vi "Init Async State Vars.vi"(8 "Error in":errorcluster, 10 "Async Parameters":T4) -> (0 "Error out":errorcluster, 3 "Async State Vars":T1)   [LabVIEW 2014, in "Waveform-Processing-Custom-Device Engine.lvlib"]
uses:
  Waveform-Processing-Custom-Device Engine.lvlib
  Types/Async Parameters.ctl
  Types/Async FIFOs.ctl
  <vilib>/NI Veristand/Custom Device API/Waveform Data Reference.ctl
  Types/Async State Vars.ctl
  <vilib>/NI Veristand/Custom Device Waveform API/Single Waveform Read (DBL)/Single Waveform Read (DBL).lvclass
  <vilib>/NI Veristand/Custom Device Waveform API/Single Waveform Write (DBL)/Single Waveform Write (DBL).lvclass
  <vilib>/NI Veristand/Custom Device API/Custom Device API.lvlib
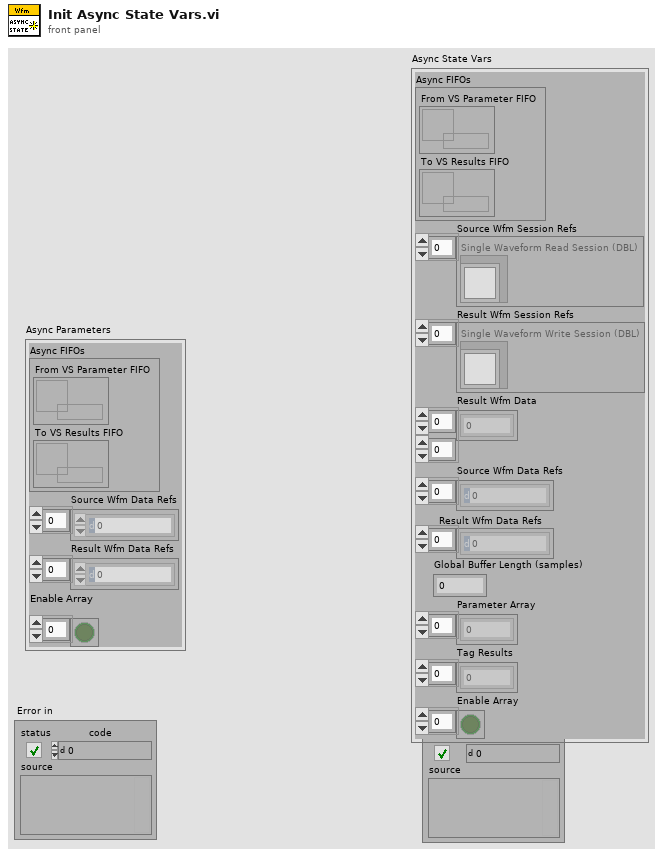
[diagram p1: front panel]
types:
  T1 = typedef "Waveform-Processing-Custom-Device Engine.lvlib/Async State Vars.ctl" = cluster{"Async FIFOs":T2, "Source Wfm Session Refs":refnum<class "Single Waveform Read (DBL).lvclass">[], "Result Wfm Session Refs":refnum<class "Single Waveform Write (DBL).lvclass">[], "Result Wfm Data":dbl[][], "Source Wfm Data Refs":T3[], "Result Wfm Data Refs":T3[], "Global Buffer Length (samples)":dbl, "Parameter Array":dbl[], "Tag Results":dbl[], "Enable Array":bool[]}
  T2 = typedef "Waveform-Processing-Custom-Device Engine.lvlib/Async FIFOs.ctl" = cluster{"From VS Parameter FIFO":refnum<k33>, "To VS Results FIFO":refnum<k33>}
  T3 = typedef "Custom Device API.lvlib/Waveform Data Reference.ctl" = i32
  T4 = typedef "Waveform-Processing-Custom-Device Engine.lvlib/Async Parameters.ctl" = cluster{"Async FIFOs":T2, "Source Wfm Data Refs":T3[], "Result Wfm Data Refs":T3[], "Enable Array":bool[]}
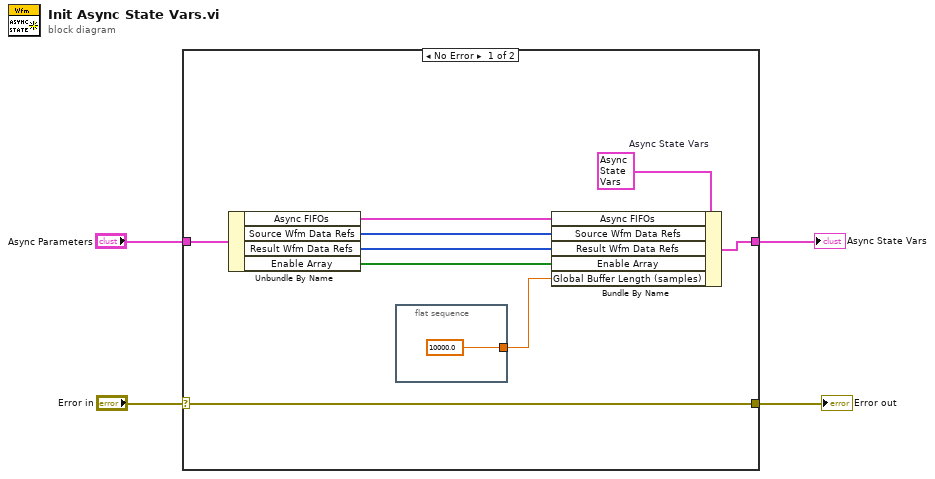
[diagram p0: block diagram]
diagram:
  n1 = case shown="No Error" "Error in" {
    selector: "Error in" -> [w7 w15]
    tunnel: [w7 w15] -> w3
    tunnel: "Async Parameters" -> [w13 _]
    tunnel: [w8 _] -> w1
    frame No Error {
      w12 = T1 {"Async FIFOs"={"From VS Parameter FIFO"=refnum, "To VS Results FIFO"=refnum}, "Source Wfm Session Refs"=[], "Result Wfm Session Refs"=[], "Result Wfm Data"=[], "Source Wfm Data Refs"=[], "Result Wfm Data Refs"=[], "Global Buffer Length (samples)"=0.0, "Parameter Array"=[], "Tag Results"=[], "Enable Array"=[]}  # Async State Vars
      n2 = Unbundle By Name(w13) -> ("Async FIFOs"=w11:T2, "Source Wfm Data Refs"=w10:T3[], "Result Wfm Data Refs"=w9:T3[], "Enable Array"=w5:bool[])
      n3 = flat-sequence {
        tunnel: [10000.0 ("Global Buffer Length (samples)")] -> w6
        frame #0 {
        }
      }
      n4 = Bundle By Name(cluster=w12, "Async FIFOs"=w11, "Source Wfm Data Refs"=w10, "Result Wfm Data Refs"=w9, "Enable Array"=w5, "Global Buffer Length (samples)"=w6) -> (w8:T1)
    }
    frame Error {
    }
  }
  "Error out" <- w3
  "Async State Vars" <- w1
